vi "Counter - Save.vi"(11 "Mode":enum16{"Reset", "Read", "Count Up"}(ring)=enum."Count Up") -> (3 "Counter":dbl)   [LabVIEW 2009]
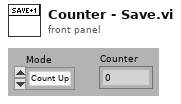
[diagram p1: front panel]
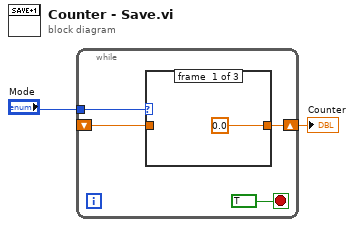
[diagram p0: block diagram]
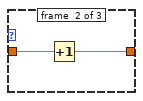
[diagram p2: hidden frame]
diagram:
  n1 = while {
    shift-right: [w6] -> w2
    shift-left: _ -> [w5]
    tunnel: "Mode" -> [w3]
    stop <- TRUE stop-if-true
    n2 = case shown="\"Count Up\", Default" w3 {
      tunnel: [0.0 w9 w10] -> w6
      tunnel: w5 -> [_ w8 w10]
      frame #0 {
      }
      frame #1 {
        n3 = Increment(x=w8) -> (x+1=w9:dbl)
      }
      frame #2 {
      }
    }
  }
  "Counter" <- w2
